vi "splashscreen.vi"() -> ()   [LabVIEW 2010]
uses:
  <vilib>/picture/picture.llb/Draw True-Color Pixmap.vi
panel:
  out "new picture":picture
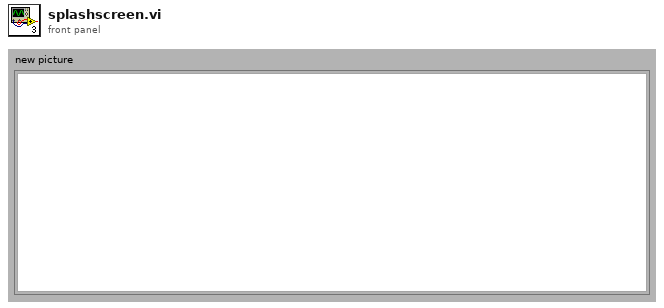
[diagram p1: front panel]
types:
  T1 = typedef "imagedata.ctl" = cluster{"image type":i32, "image depth":i32, "image":u8[], "mask":u8[], "colors":u32[], "Rectangle":cluster{"left":i16, "top":i16, "right":i16, "bottom":i16}}
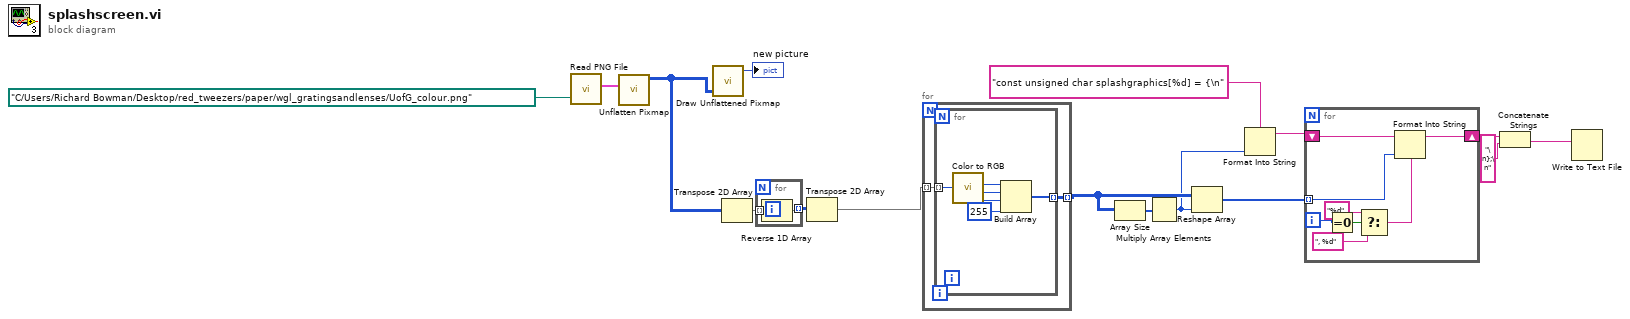
[diagram p0: block diagram]
diagram:
  n1 = call <vilib>:"Read PNG File.vi"("path to PNG file"=path "C:/Users/Richard Bowman/Desktop/red_tweezers/paper/wgl_gratingsandlenses/UofG_colour.png") -> ("image data"=w16:T1)  [unwired: 8 in, 2 out]
  n2 = call <vilib>:"Unflatten Pixmap.vi"("image data"=w16) -> ("24-bit pixmap"=w11:u32[][])  [unwired: 4 in, 6 out]
  n3 = call-poly <vilib>:"Draw Unflattened Pixmap.vi"("data (RGB format)"=w11) -> ("new picture"=→"new picture":picture)  [unwired: 8 in]
  n4 = Transpose 2D Array(2D array=w11) -> (transposed array=w13:u32[][])
  n5 = for {
    tunnel: w13 -> [w18] mode=indexing
    tunnel: [w17] -> w12 mode=indexing
    n6 = Reverse 1D Array(array=w18) -> (reversed array=w17:u32[])
  }
  n7 = Transpose 2D Array(2D array=w12) -> (transposed array=w9:u32[][])
  n8 = for {
    tunnel: w9 -> [w19] mode=indexing
    tunnel: [w20] -> w8 mode=indexing
    n9 = for {
      tunnel: w19 -> [w26] mode=indexing
      tunnel: [w21] -> w20 mode=indexing
      n10 = call <vilib>:"Color to RGB.vi"("Color"=w26) -> ("R"=w23:u8, "G"=w25:u8, "B"=w24:u8)  [unwired: 1 out]
      n11 = Build Array(w23, w25, w24, u8 255 ("element")) -> (w21:u8[])
    }
  }
  n12 = Array Size(array=w8) -> (size(s)=w10:i32[])
  n13 = Multiply Array Elements(1:w10) -> (0:w6:i32)
  n14 = Reshape Array(w8, w6) -> (w5:u8[])
  n15 = Format Into String(format string="const unsigned char splashgraphics[%d] = {\n", w6) -> (resulting string=w4:string)  [unwired: 2 in, 1 out]
  n16 = for {
    tunnel: w5 -> [w34] mode=indexing
    shift-right: [w32] -> w3
    shift-left: w4 -> [w33]
    i -> [w31]
    n17 = Equal To 0?(x=w31) -> (x = 0?=w30:bool)
    n18 = Select(t="%d" ("format string"), s=w30, f=", %d") -> (s? t:f=w27:string)
    n19 = Format Into String(format string=w27, initial string=w33, w34) -> (resulting string=w32:string)  [unwired: 1 in, 1 out]
  }
  n20 = Concatenate Strings(w3, "\n};\n" ("string")) -> (w1:string)
  n21 = Write to Text File(text=w1) -> ()  [unwired: 3 in, 3 out]
